vi "main.vi"(8 "Error in":errorcluster) -> (0 "Error out":errorcluster)   [LabVIEW 2018, in "template.lvlib"]
uses:
  template.lvlib
  modules/Common/Common.lvlib
  ctl/Module Queue - Action.ctl
  ctl/Module - State.ctl
  modules/Common/ctl/Stop All - Action.ctl
  modules/Error Handler/Error Handler.lvlib
  modules/Error Handler/ctl/Module - State.ctl
  modules/Controller/Controller.lvlib
  modules/Controller/ctl/Module - State.ctl
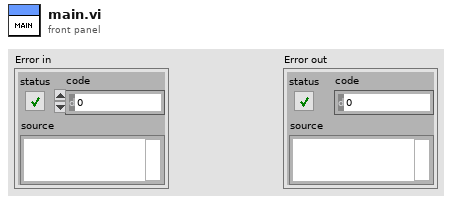
[diagram p1: front panel]
types:
  T1 = typedef "template.lvlib/Module Queue - Action.ctl" = enum16{"Create", "Get", "Destroy"}
  T2 = typedef "Common.lvlib/Stop All - Action.ctl" = enum16{"Create", "Fire", "Get", "Destroy"}
  T3 = typedef "template.lvlib/Module - State.ctl" = enum16{"Init", "Idle", "Error", "Close"}
  T4 = typedef "Controller.lvlib/Module - State.ctl" = enum16{"Init", "Idle", "Error", "Close"}
  T5 = typedef "Error Handler.lvlib/Module - State.ctl" = enum16{"Init", "Idle", "Error", "Close", "Handle External Error", "Log Error"}
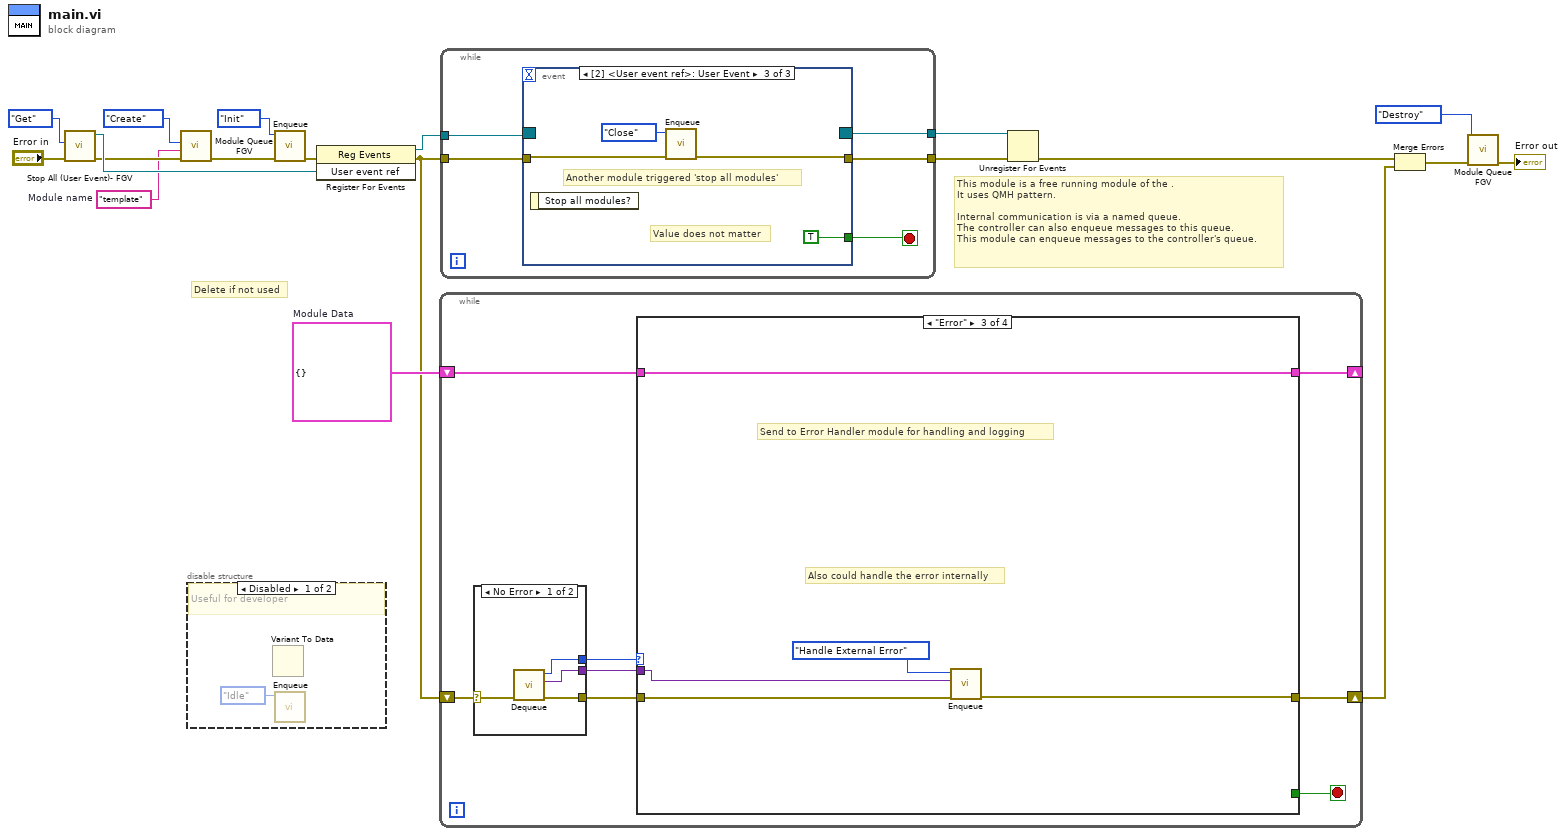
[diagram p0: block diagram]
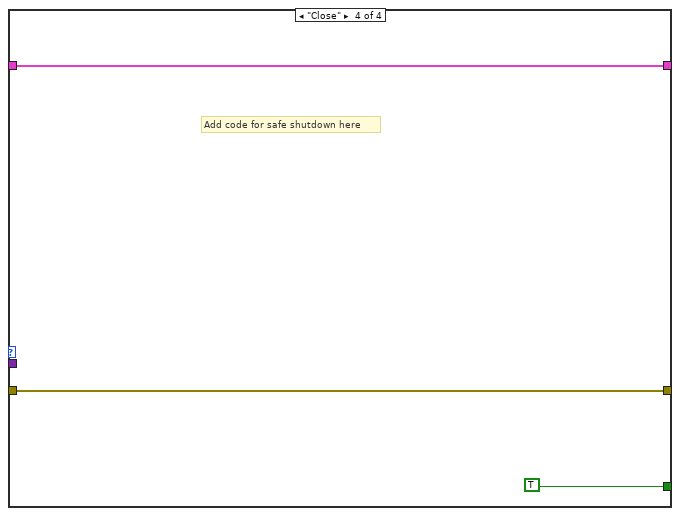
[diagram p4: hidden frame]
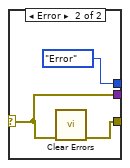
[diagram p5: hidden frame]
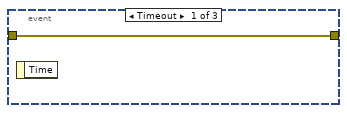
[diagram p7: hidden frame]
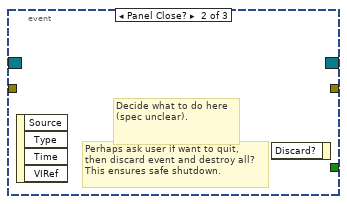
[diagram p8: hidden frame]
diagram:
  w1 = "template"  # Module name
  w8 = cluster{} {}  # Module Data
  # "This module is a free running module of the .\nIt uses QMH pattern.\n\nInternal communication is via a named queue.\nThe controller can also enqueue messages to this queue.\nThis module can enqueue messages to the controller's queue."
  # "Delete if not used"
  n1 = call "Stop All (User Event)- FGV.vi"("error in"="Error in", "Action"=Stop_All_-_Action."Get") -> ("error out"=w10:errorcluster, "User event ref"=w15:refnum<user-event>)  [unwired: 8 in]
  n2 = call "Module Queue FGV.vi"("Error in"=w10, "Queue name"=w1, "Action"=Module_Queue_-_Action."Create") -> ("Error out"=w18:errorcluster)  [unwired: 7 in, 1 out]
  n3 = disable-structure shown="Disabled" {
    frame Disabled {
      # "Useful for developer"
      n4 = Variant To Data() -> ()  [unwired: 3 in, 2 out]
      n5 = call "Enqueue.vi"("State"=Module_-_State."Idle") -> ()  [unwired: 10 in, 1 out]
    }
    frame Enabled {
    }
  }
  n6 = call "Enqueue.vi"("error in (no error)"=w18, "State"=Module_-_State."Init") -> ("error out"=w9:errorcluster)  [unwired: 9 in]
  n7 = register-events(error in=w9, w15) -> (reference out=w13:refnum<event-registration>, error out=w3:errorcluster)  [unwired: 1 in]
  n8 = while {
    shift-right: [w28] -> _
    shift-left: w8 -> [w27]
    shift-right: [w21] -> w2
    shift-left: w3 -> [w26]
    stop <- w22 stop-if-true
    n9 = case shown="No Error" w26 {
      selector: w26 -> [w43 w45]
      tunnel: [w42 Module_-_State."Error" ("State")] -> w25
      tunnel: [w41 w45] -> w24
      tunnel: [w40 w44] -> w23
      frame No Error {
        n10 = call "Dequeue.vi"("error in"=w43) -> ("error out"=w40:errorcluster, "Data"=w41:variant, "State"=w42:T3)  [unwired: 8 in]
      }
      frame Error {
        # "Instead of dequeue,\nhandle the error"
        n11 = call <vilib>:"Clear Errors.vi"("error in (no error)"=w45) -> ("error out"=w44:errorcluster)  [unwired: 5 in, 1 out]
      }
    }
    n12 = case shown="\"Error\"" w25 {
      tunnel: [w29 w31 w36 w37] -> w28
      tunnel: w27 -> [w29 w31 w36 w37]
      tunnel: w24 -> [_ _ w33 _]
      tunnel: w23 -> [_ w30 w35 w38]
      tunnel: [_ _ _ TRUE] -> w22
      tunnel: [_ w30 w34 w38] -> w21
      frame "Init", Default {
      }
      frame "Idle" {
      }
      frame "Error" {
        # "Send to Error Handler module for handling and logging"
        # "Also could handle the error internally"
        n13 = call "Enqueue.vi"("error in (no error)"=w35, "Data"=w33, "State"=Module_-_State."Handle External Error") -> ("error out"=w34:errorcluster)  [unwired: 8 in]
      }
      frame "Close" {
        # "Add code for safe shutdown here"
      }
    }
  }
  n14 = while {
    tunnel: w13 -> [w51]
    tunnel: [w50] -> w12
    tunnel: w3 -> [w49]
    tunnel: [w48] -> w11
    stop <- w47 stop-if-true
    n15 = event shown="[2] <User event ref>: User Event" {
      selector: w51 -> [_ _ _]
      dyn-events: [_ _ _] -> w50
      timeout: _ -> [_ _ _]
      tunnel: w49 -> [w52 _ w56]
      tunnel: [w52 _ w55] -> w48
      tunnel: [_ _ TRUE] -> w47
      event Timeout {
        n16 = event-data() -> ()  [unwired: 1 in, 1 out]
      }
      event Panel Close? {
        # "Perhaps ask user if want to quit,\nthen discard event and destroy all?\nThis ensures safe shutdown."
        # "Decide what to do here\n(spec unclear)."
        n17 = event-data() -> ()  [unwired: 1 in, 4 out]
        n18 = event-data() -> ()  [unwired: 2 in, 1 out]
      }
      event User Event {
        # "Value does not matter"
        # "Another module triggered 'stop all modules'"
        n19 = event-data() -> ()  [unwired: 1 in, 1 out]
        n20 = call "Enqueue.vi"("error in (no error)"=w56, "State"=Module_-_State."Close") -> ("error out"=w55:errorcluster)  [unwired: 9 in]
      }
    }
  }
  n21 = Unregister For Events(event registration refnum=w12, error in=w11) -> (error out=w7:errorcluster)
  n22 = Merge Errors(w7, w2) -> (w6:errorcluster)
  n23 = call "Module Queue FGV.vi"("Error in"=w6, "Action"=Module_Queue_-_Action."Destroy") -> ("Error out"=→"Error out":errorcluster)  [unwired: 8 in, 1 out]
